vi "readFromXML.vi"(8 "error in (no error)":errorcluster, 10 "XML in":string, 11 "TCSMCCCommand in":refnum<class "TCSMCCCommand.lvclass">) -> (0 "error out":errorcluster, 3 "TCSMCCCommand out":refnum<class "TCSMCCCommand.lvclass">)   [LabVIEW 2022 SP3, in "TCSDataDefinitions.lvlib" / "TCSMountControlCommand.lvlib" / "TCSMCCCommand.lvclass"]
uses:
  TCSMCCCommand.lvclass
  TCSCommand/TCSCommand/TCSCommand.lvclass
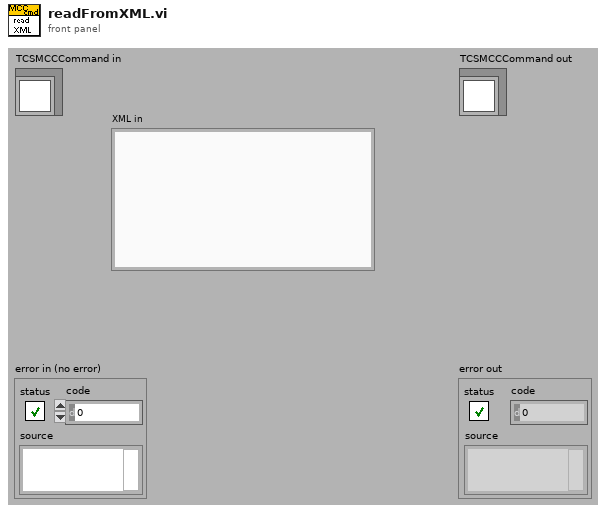
[diagram p1: front panel]
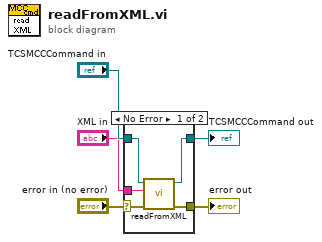
[diagram p0: block diagram]
diagram:
  n1 = case shown="No Error" "error in (no error)" {
    selector: "error in (no error)" -> [w7 w11]
    tunnel: [w6 w11] -> w4
    tunnel: [w8 w12] -> w2
    tunnel: "TCSMCCCommand in" -> [w9 w12]
    tunnel: "XML in" -> [w10 _]
    frame No Error {
      n2 = call-parent "readFromXML.vi"("error in (no error)"=w7, "XML in"=w10, "TCSCommand in"=w9) -> ("error out"=w6:errorcluster, "TCSCommand out"=w8:refnum<class "TCSMCCCommand.lvclass">)  [unwired: 7 in]
    }
    frame Error {
    }
  }
  "error out" <- w4
  "TCSMCCCommand out" <- w2
